vi "Getlimit.vi"(8 "error in (no error)":errorcluster, 11 "B&K Precision 9120 series in":refnum<class "B&K Precision 9120 series.lvclass">) -> (0 "error out":errorcluster, 1 "Current read":dbl, 2 "Voltage read":dbl, 3 "B&K Precision 9120 series out":refnum<class "B&K Precision 9120 series.lvclass">)   [LabVIEW 2014, in "B&K Precision 9120 series.lvclass"]
uses:
  B&K Precision 9120 series.lvclass
  B&K Precision 9120 series.lvclass/B&K Precision 9120 series.ctl
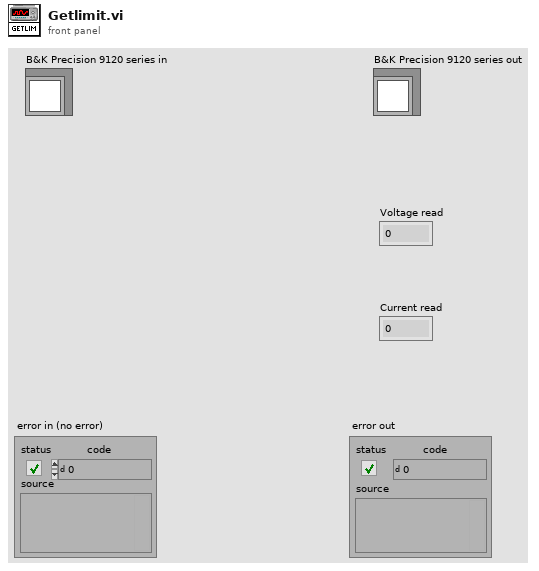
[diagram p1: front panel]
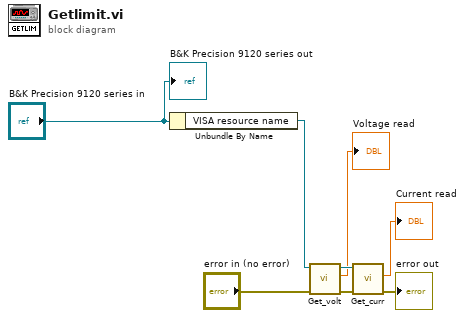
[diagram p0: block diagram]
diagram:
  n1 = Unbundle By Name("B&K Precision 9120 series in") -> ("VISA resource name"=w2:refnum<visa-resource-name>)
  n2 = call "Get_volt.vi"("error in (no error)"="error in (no error)", "VISA resource in"=w2) -> ("error out"=w6:errorcluster, "voltage"=→"Voltage read":dbl, "VISA resource out"=w7:refnum<visa-resource-name>)  [unwired: 7 in]
  n3 = call "Get_curr.vi"("error in (no error)"=w6, "VISA resource in"=w7) -> ("error out"=→"error out":errorcluster, "current"=→"Current read":dbl)  [unwired: 7 in, 1 out]
  "B&K Precision 9120 series out" <- "B&K Precision 9120 series in"
